vi "Is valid.vi"(11 "address":refnum<class "IPv4 Network Address.lvclass">) -> (2 "valid?":bool, 3 "address out":refnum<class "IPv4 Network Address.lvclass">)   [LabVIEW 2020, in "NI_WFCN.lvlib" / "IPv4 Network Address.lvclass"]
doc: "Does this object actually store a network address? (If FALSE, this object is just a stub.)"
uses:
  <vilib>/net/WFCN/Addressing/IPv4 Network Address/IPv4 Network Address.lvclass
  <vilib>/net/WFCN/Addressing/IPv4 Network Address/IPv4 Network Address.lvclass/IPv4 Network Address.ctl
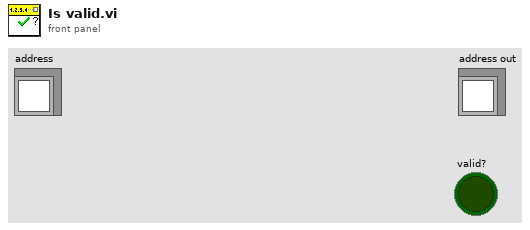
[diagram p1: front panel]
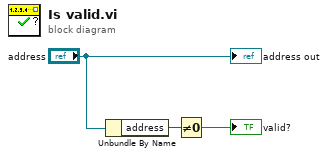
[diagram p0: block diagram]
diagram:
  n1 = Unbundle By Name("address") -> ("address"=w2:u32)
  n2 = Not Equal To 0?(x=w2) -> (x != 0?=→"valid?":bool)
  "address out" <- "address"
